vi "DHE_GetNumberFromName.vi"(8 "error in (no error)":errorcluster, 11 "Database RefNum in":T1) -> (0 "error out":errorcluster, 1 "lastimg":string, 2 "number":u16)   [LabVIEW 2016]
uses:
  DBSHAND/private/vis/DatabaseHand_RefNum.ctl
  DBSHAND/private/vis/DatabaseHand_Element_Get(string).vi
  DBSHAND/private/vis/DatabaseHand_Element_Get(U16).vi
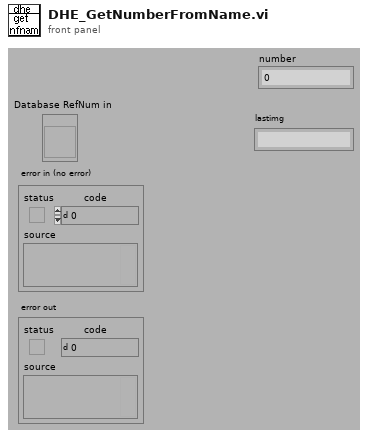
[diagram p1: front panel]
types:
  T1 = typedef "DatabaseHand_RefNum.ctl" = refnum<vi>
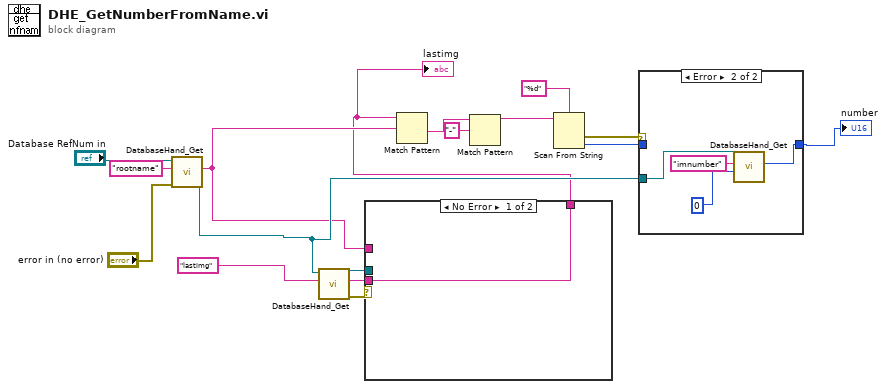
[diagram p0: block diagram]
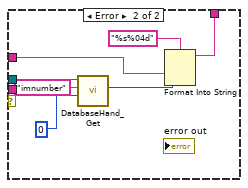
[diagram p3: hidden frame]
diagram:
  n1 = call-poly "DatabaseHand_Get.vi"("error in (no error)"="error in (no error)", "name"="rootname", "Database RefNum in"="Database RefNum in") -> ("value"=w3:string, "Database RefNum out"=w5:T1)  [unwired: 2 in, 5 out]
  n2 = call-poly "DatabaseHand_Get.vi"("name"="lastimg", "Database RefNum in"=w5) -> ("error out"=w14:errorcluster, "value"=w12:string, "Database RefNum out"=w13:T1)  [unwired: 3 in, 4 out]
  n3 = case shown="No Error" w14 {
    tunnel: w13 -> [_ w25]
    tunnel: w3 -> [_ w22]
    tunnel: [w18 w19] -> w1
    tunnel: w12 -> [w18 _]
    frame No Error {
    }
    frame Error {
      n4 = call-poly "DatabaseHand_Get.vi"("default value"=u16 0 ("number"), "name"="imnumber", "Database RefNum in"=w25) -> ("value"=w21:u16)  [unwired: 2 in, 6 out]
      n5 = Format Into String(format string="%s%04d", w22, w21) -> (resulting string=w19:string)  [unwired: 2 in, 1 out]
    }
  }
  "lastimg" <- w1
  n6 = Match Pattern(string=w1, regular expression=w3) -> (after substring=w11:string)  [unwired: 4 out]
  n7 = Match Pattern(string=w11, regular expression="-") -> (before substring=w9:string)  [unwired: 4 out]
  n8 = Scan From String(format string="%d", input string=w9) -> (error out=w7:errorcluster, output 1=w6:i32)  [unwired: 2 in, 3 out]
  n9 = case shown="Error" w7 {
    tunnel: w6 -> [w26 _]
    tunnel: w5 -> [_ w28]
    tunnel: [w26 w27] -> w4
    frame No Error {
    }
    frame Error {
      n10 = call-poly "DatabaseHand_Get.vi"("default value"=u16 0 ("number"), "name"="imnumber", "Database RefNum in"=w28) -> ("value"=w27:u16)  [unwired: 2 in, 6 out]
    }
  }
  "number" <- w4
